vi "ExSpectSetMirrorPos.vi"() -> ()   [LabVIEW 2010]
panel:
  in  "Mirror Number":i16=1 min=1 max=4 step=1
  in  "Position":i16=1 min=1 max=2 step=1
  out "error out":errorcluster
  in  "error in (no error)":errorcluster
  # "ExSpectSetMirrorPos.vi\n(Normal Spectrograph via USB/COM port)\nThis VI will set the selected mirror to the selected position.."
  # "NOTES:\nA properly configured spectometer .ini must be present in the LabVIEW folder for spectrograph operation.\n\nConsult the Toolkit documentation for more information on how to configure this file."
  # "1 = Entrance\n 2 = Exit"
  # "1 = Front\n 2 = Side"
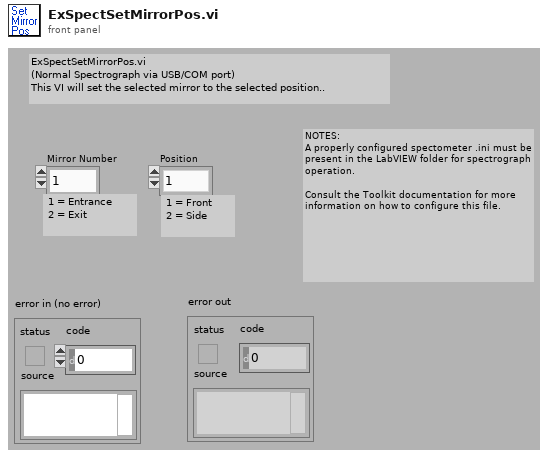
[diagram p1: front panel]
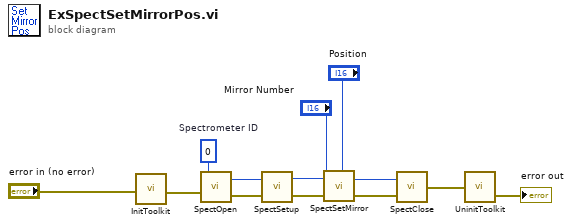
[diagram p0: block diagram]
diagram:
  w11 = u32 0  # Spectrometer ID
  n1 = call <userlib>:"InitToolkit.vi"("error in"="error in (no error)") -> ("error out"=w8:errorcluster)
  n2 = call <userlib>:"SpectOpen.vi"("error in"=w8, "Spectrometer ID"=w11) -> ("error out"=w12:errorcluster, "Spectrometer Handle"=w13:u32)  [unwired: 1 in]
  n3 = call <userlib>:"SpectSetup.vi"("error in"=w12, "Spectrometer Handle"=w13) -> ("error out"=w7:errorcluster, "Spectrometer Handle"=w4:u32)
  n4 = call <userlib>:"SpectSetMirror.vi"("error in"=w7, "Position"="Position", "Mirror"="Mirror Number", "Spectrometer Handle"=w4) -> ("error out"=w6:errorcluster, "Spectrometer Handle"=w5:u32)
  n5 = call <userlib>:"SpectClose.vi"("error in"=w6, "Spectrometer Handle"=w5) -> ("error out"=w1:errorcluster)
  n6 = call <userlib>:"UninitToolkit.vi"("error in"=w1) -> ("error out"=→"error out":errorcluster)
